vi "BB_Testing.vi"() -> ()   [LabVIEW 2012]
uses:
  BotSpeakSubs/BotspeakSettingsUsed.vi
  SubVIs/LVPresent_Globals.vi
panel:
  in  "LED3":bool
  in  "LED1":bool
  in  "LED2":bool
  in  "LED0":bool
  # "Test the BeagleBoard\n\nTry clicking the buttons below to turn on the user LEDs on the BeagleBoard."
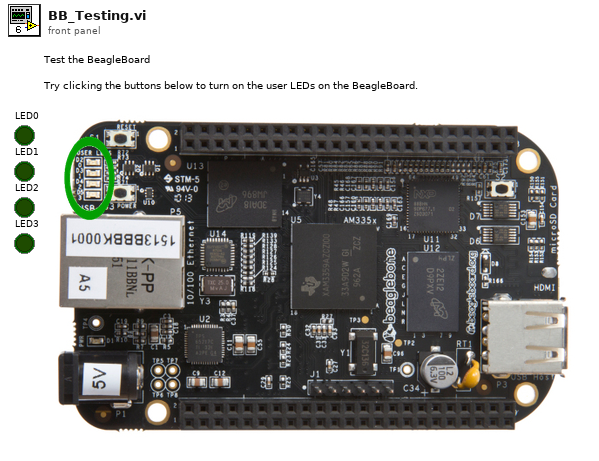
[diagram p1: front panel]
types:
  T1 = typedef "BotSpeak_Control.ctl" = cluster{"Address":string, "Reply EOF":string, "Hardware":string, "Retries":i8, "Timeout":i32}
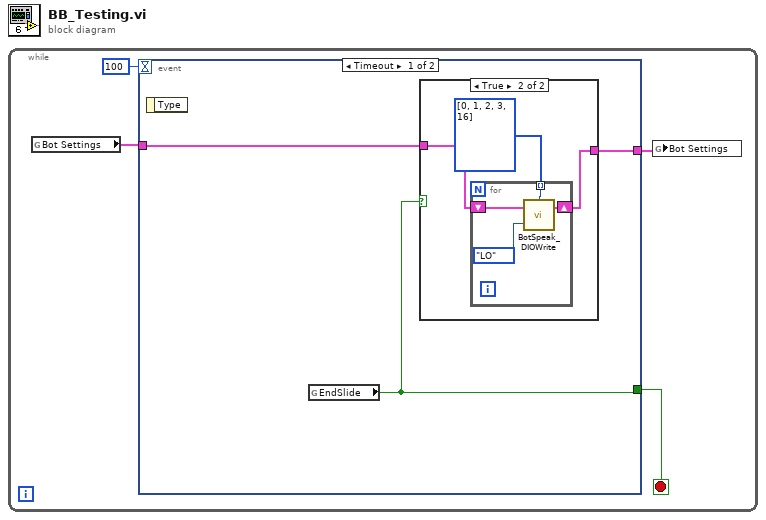
[diagram p0: block diagram]
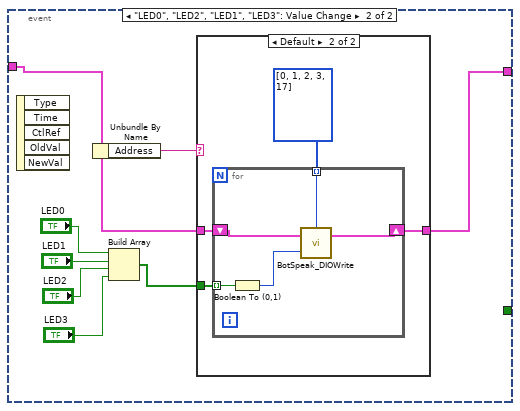
[diagram p3: hidden frame]
diagram:
  n1 = while {
    stop <- w4 stop-if-true
    n2 = global read "BotspeakSettingsUsed.vi" "Bot Settings"() -> (w2:T1)
    n3 = event shown="[0] Timeout" {
      selector: _ -> [_ _]
      dyn-events: _ -> [_ _]
      timeout: 100 -> [_ _]
      tunnel: [w7 _] -> w4
      tunnel: w2 -> [w6 w18]
      tunnel: [w5 w19] -> w1
      event Timeout {
        n4 = event-data() -> ()  [unwired: 1 in, 1 out]
        n5 = global read "LVPresent_Globals.vi" "EndSlide"() -> (w7:bool)
        n6 = case shown="True" w7 {
          tunnel: w6 -> [w8 w10]
          tunnel: [w8 w9] -> w5
          frame False {
          }
          frame True {
            n7 = for {
              tunnel: i32[] [0, 1, 2, 3, 16] -> [w15] mode=indexing
              shift-right: [w12] -> w9
              shift-left: w10 -> [w13]
              n8 = call <userlib>:"BotSpeak_DIOWrite.vi"("State"=enum32{"LO", "HI"}."LO", "Bot Settings"=w13, "DIO Line"=w15) -> ("Bot Settings"=w12:T1)  [unwired: 1 out]
            }
          }
        }
      }
      event "LED0", "LED2", "LED1", "LED3": Value Change {
        n9 = event-data() -> ()  [unwired: 1 in, 5 out]
        n10 = Unbundle By Name(w18) -> ("Address"=w17:string)
        n11 = Build Array("LED0", "LED1", "LED2", "LED3") -> (w20:bool[])
        n12 = case shown="Default" w17 {
          tunnel: w20 -> [_ w27]
          tunnel: w18 -> [w24 w26]
          tunnel: [w24 w25] -> w19
          frame "" {
          }
          frame Default {
            n13 = for {
              tunnel: i32[] [0, 1, 2, 3, 17] ("Array") -> [w32] mode=indexing
              tunnel: w27 -> [w31] mode=indexing
              shift-right: [w29] -> w25
              shift-left: w26 -> [w30]
              n14 = Boolean To (0,1)(Boolean=w31) -> (0, 1=w33:i16)
              n15 = call <userlib>:"BotSpeak_DIOWrite.vi"("State"=w33, "Bot Settings"=w30, "DIO Line"=w32) -> ("Bot Settings"=w29:T1)  [unwired: 1 out]
            }
          }
        }
      }
    }
    n16 = global write "BotspeakSettingsUsed.vi" "Bot Settings"(w1) -> ()
  }
